vi "Read_Traverse_Pos_File.vi"(1 "Traverse Name":string="EnFlo Tunnel") -> (0 "Tunnel Coordinates":sgl[](array[numeric]) format="%.2f")   [LabVIEW 2014]
uses:
  ADAM Serial/Instrument drivers/Traverses/~subVIs/AxisConfigCluster.ctl
  ADAM Serial/Instrument drivers/Traverses/~subVIs/DriveProperties.ctl
  ADAM Serial/Instrument drivers/Traverses/~subVIs/DriveStaticConfig.ctl
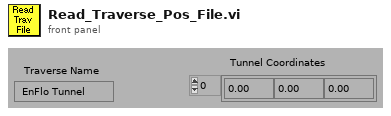
[diagram p1: front panel]
types:
  T1 = typedef "AxisConfigCluster.ctl" = cluster{"Channel Properties":T2, "Static Drive Configuration":T3}
  T2 = typedef "DriveProperties.ctl" = cluster{"Channel Name":string, "Vel. Default":sgl, "Acc. Default":sgl, "Vel. Max":sgl, "Vel. Min":sgl, "Acc. Max":sgl, "Acc. Min":sgl, "Pulses/unit":sgl, "Address":u8, "Pulse Offset":i32, "Pos Tolerance":sgl, "Pulses/rev":sgl, "Backlash/Eng units":sgl, "Current Pos":sgl, "Ch Status":enum16{"Active", "Offline", "Simulate"}, "Port Name":string, "Axis Transform mode":string, "Metadata Ch Name":string, "Type":string}
  T3 = typedef "DriveStaticConfig.ctl" = cluster{"Correction Gain % (CG)":u16, "Dead Band (DB)":i32, "Dead Band Window (DW)":i32, "Encoder Resolution (ER)":i32, "Step Mode  (FSB)":u16, "Position Maintenance (FSC)":u16, "Stop on Stall (FSD)":u16, "Activate OP1 on stall (FSE)":u16, "Stop on Trigger 3 (FSF)":u16, "OP2 in Deadband (FSG)":u16, "Stall Detect (FSH)":u16, "Limit Disable (LD)":u16, "Motor Resolution (MR)":enum16{"200", "400", "1000", "2000", "4000", "5000", "10000", "12800", "18000", "20000", "21600", "25000", "25400", "25600", "36000", "50000", "278528", "425984", "507904", "614400", "655360", "819200", "1024000"}, "Limit Switch Sense (OSA)":u16, "Home Position (OSB)":u16, "Home Switch Sense (OSC)":u16, "Encoder Z for Home (OSD)":u16, "Reference edge of Home (OSH)":u16, "RS232 Echo Control (SSA)":u16, "Buffer at Limit (SSG)":u16, "Buffer at Stop (SSH)":u16, "Indexer Mode  (FSA)":u16, "Type":string, "ConfigString":string, "De Power Motor":enum16{"TRUE", "FALSE"}}
  T4 = enum16{"Load setup from excel file", "Save setup to excel file"}
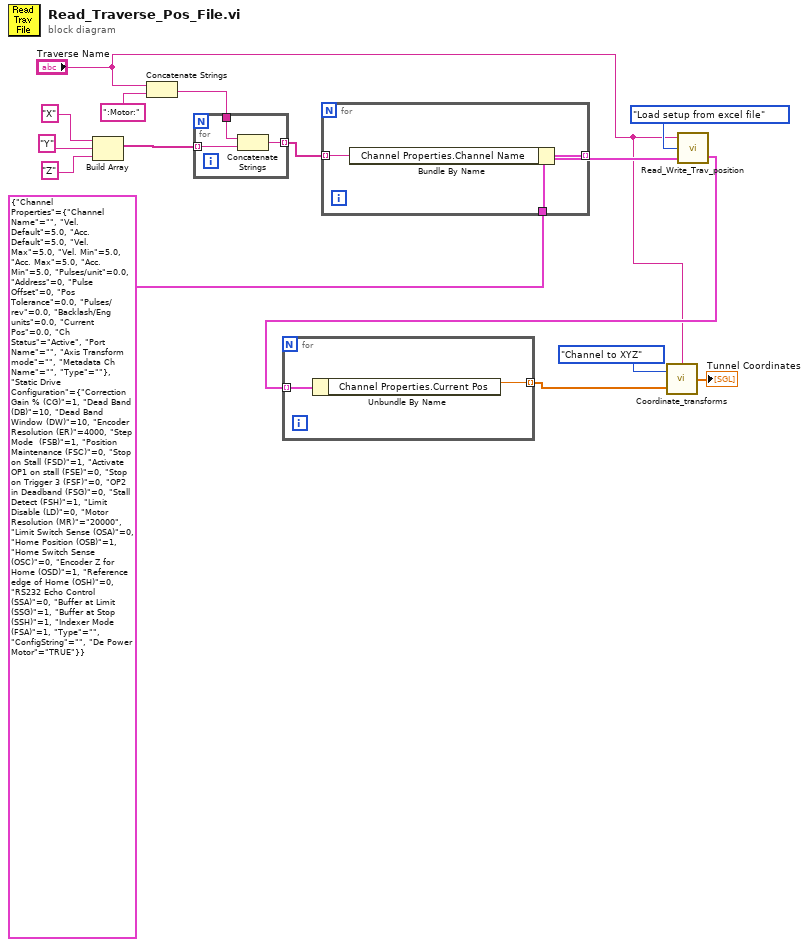
[diagram p0: block diagram]
diagram:
  n1 = Build Array("X", "Y", "Z") -> (w11:string[])
  n2 = Concatenate Strings("Traverse Name", ":Motor:") -> (w12:string)
  n3 = for {
    tunnel: w11 -> [w18] mode=indexing
    tunnel: [w16] -> w7 mode=indexing
    tunnel: w12 -> [w17]
    n4 = Concatenate Strings(w17, w18) -> (w16:string)
  }
  n5 = for {
    tunnel: [w21] -> w6 mode=indexing
    tunnel: T1 {"Channel Properties"={"Channel Name"="", "Vel. Default"=5.0, "Acc. Default"=5.0, "Vel. Max"=5.0, "Vel. Min"=5.0, "Acc. Max"=5.0, "Acc. Min"=5.0, "Pulses/unit"=0.0, "Address"=0, "Pulse Offset"=0, "Pos Tolerance"=0.0, "Pulses/rev"=0.0, "Backlash/Eng units"=0.0, "Current Pos"=0.0, "Ch Status"=enum."Active", "Port Name"="", "Axis Transform mode"="", "Metadata Ch Name"="", "Type"=""}, "Static Drive Configuration"={"Correction Gain % (CG)"=1, "Dead Band (DB)"=10, "Dead Band Window (DW)"=10, "Encoder Resolution (ER)"=4000, "Step Mode  (FSB)"=1, "Position Maintenance (FSC)"=0, "Stop on Stall (FSD)"=1, "Activate OP1 on stall (FSE)"=0, "Stop on Trigger 3 (FSF)"=0, "OP2 in Deadband (FSG)"=0, "Stall Detect (FSH)"=1, "Limit Disable (LD)"=0, "Motor Resolution (MR)"=enum."20000", "Limit Switch Sense (OSA)"=0, "Home Position (OSB)"=1, "Home Switch Sense (OSC)"=0, "Encoder Z for Home (OSD)"=1, "Reference edge of Home (OSH)"=0, "RS232 Echo Control (SSA)"=0, "Buffer at Limit (SSG)"=1, "Buffer at Stop (SSH)"=1, "Indexer Mode  (FSA)"=1, "Type"="", "ConfigString"="", "De Power Motor"=enum."TRUE"}} ("Channel Description") -> [w20]
    tunnel: w7 -> [w19] mode=indexing
    n6 = Bundle By Name(cluster=w20, "Channel Properties.Channel Name"=w19) -> (w21:T1)
  }
  n7 = call "Read_Write_Trav_position.vi"("Matched Configurations In"=w6, "Mode"=T4."Load setup from excel file", "Traverse Name"="Traverse Name") -> ("Matched Configurations Out"=w5:T1[])  [unwired: 1 out]
  n8 = for {
    tunnel: [w23] -> w3 mode=indexing
    tunnel: w5 -> [w22] mode=indexing
    n9 = Unbundle By Name(w22) -> ("Channel Properties.Current Pos"=w23:sgl)
  }
  n10 = call "Coordinate_transforms.vi"("Traverse Name"="Traverse Name", "Input"=w3, "Mode"=enum16{"XYZ to Channel", "Channel to XYZ"}."Channel to XYZ") -> ("Output"=→"Tunnel Coordinates":sgl[])
